vi "StopSubroutine.vi"(8 "error in (no error)":errorcluster, 11 "AutoSubroutine in":refnum<class "AutoSubroutine.lvclass">) -> (0 "error out":errorcluster, 2 "Stop Loop?":bool, 3 "AutoSubroutine out":refnum<class "AutoSubroutine.lvclass">)   [LabVIEW 2017, in "AutoSubroutine.lvclass"]
uses:
  AutoSubroutine.lvclass
  AutoSubroutine.lvclass/AutoSubroutine.ctl
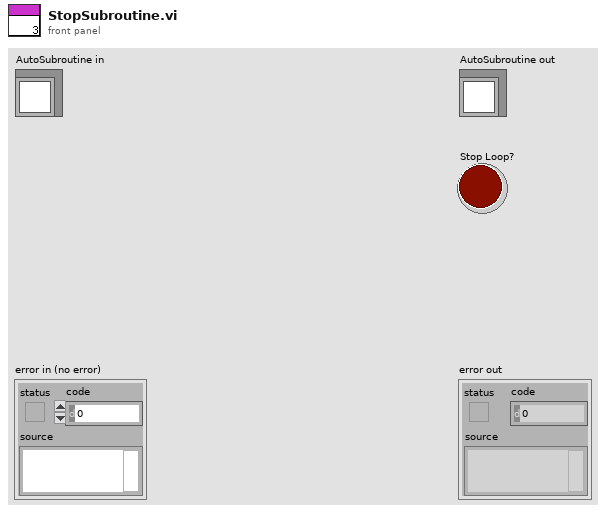
[diagram p1: front panel]
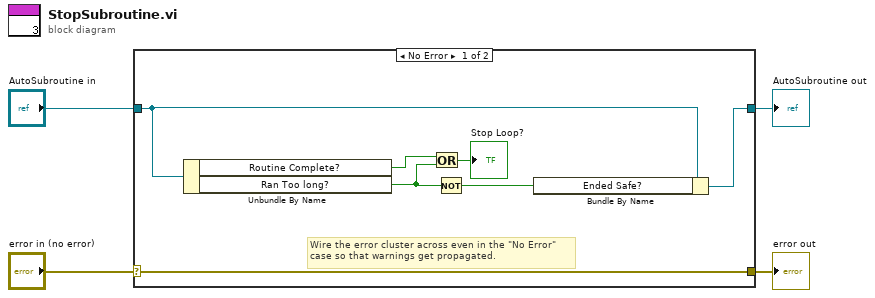
[diagram p0: block diagram]
diagram:
  n1 = case shown="No Error" "error in (no error)" {
    selector: "error in (no error)" -> [w11 w13]
    tunnel: [w11 w13] -> w3
    tunnel: [w9 w12] -> w1
    tunnel: "AutoSubroutine in" -> [w7 w12]
    frame No Error {
      # "Wire the error cluster across even in the \"No Error\"\ncase so that warnings get propagated."
      n2 = Unbundle By Name(w7) -> ("Routine Complete?"=w5:bool, "Ran Too long?"=w6:bool)
      n3 = Or(x=w5, y=w6) -> (x .or. y?=→"Stop Loop?":bool)
      n4 = Not(x=w6) -> (.not. x?=w8:bool)
      n5 = Bundle By Name(cluster=w7, "Ended Safe?"=w8) -> (w9:refnum<class "AutoSubroutine.lvclass">)
    }
    frame Error {
    }
  }
  "error out" <- w3
  "AutoSubroutine out" <- w1
